vi "event start stop flow test.vi"() -> ()   [LabVIEW 2010]
panel:
  out "little it":dbl
  out "big it":dbl
  in  "Start Run":bool caption="Make all inputs are set before hitting start!!!"
  in  "stop":bool
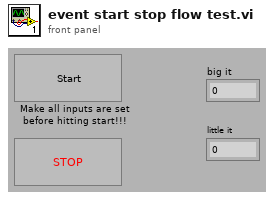
[diagram p1: front panel]
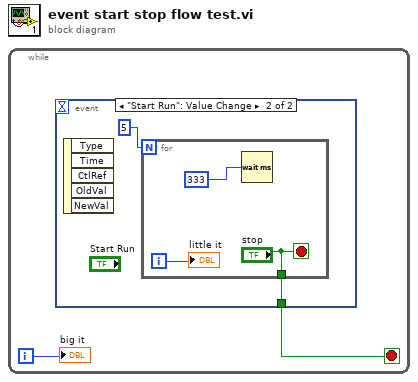
[diagram p0: block diagram]
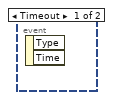
[diagram p2: hidden frame]
diagram:
  n1 = while {
    i -> [w2]
    stop <- w1 stop-if-true
    n2 = event shown="[1] \"Start Run\": Value Change" {
      selector: _ -> [_ _]
      dyn-events: _ -> [_ _]
      timeout: _ -> [_ _]
      tunnel: [_ w4] -> w1
      event Timeout {
        n3 = event-data() -> ()  [unwired: 1 in, 2 out]
      }
      event "Start Run": Value Change {
        n4 = event-data() -> ()  [unwired: 1 in, 5 out]
        n5 = for {
          N: 5 -> [_]
          tunnel: ["stop"] -> w4
          i -> [w7]
          stop <- "stop" stop-if-true
          n6 = Wait (ms)(milliseconds to wait=333) -> ()  [unwired: 1 out]
          "little it" <- w7
        }
      }
    }
    "big it" <- w2
  }
